vi "For Testing.vi"() -> ()   [LabVIEW 2018]
uses:
  <vilib>/DAQmx/write.llb/DAQmx Write (Analog DBL 1Chan 1Samp).vi
  <vilib>/DAQmx/read.llb/DAQmx Read (Analog DBL 1Chan 1Samp).vi
  <vilib>/addons/control/pid/pid.llb/PID Gain Schedule (DBL).vi
  <vilib>/addons/control/pid/pid.llb/PID Advanced (DBL).vi
  <vilib>/DAQmx/create/channels.llb/DAQmx Create Channel (AI-Voltage-Basic).vi
  <vilib>/DAQmx/miscellaneous.llb/DAQmx Fill In Error Info.vi
  <vilib>/addons/control/pid/NI_PID_pid.lvlib
panel:
  out "Pressure (in torr)":dbl
  out "Scaled MV":dbl(slide) scale=0.0..2000.0
  in  "stop":bool
  out "Preessure Readout":dbl(knob) scale=0.0..1000.0
  in  "Target pressure":dbl
  in  "Sampling Time dt (s)":dbl=0.05 min=0.001 step=0.01 format="%#.3p"
  in  "PID gain schedule":T1(array[cluster])=[{"PID gains"={"proportional gain (Kc)"=1.0, "integral time (Ti, min)"=0.01, "derivative time (Td, min)"=0.0}, "max value"=100.0}] {"max value" format="%.2f"; "PID gains"."derivative time (Td, min)" format="%.6f"; "PID gains"."integral time (Ti, min)" format="%.6f"; "PID gains"."proportional gain (Kc)" format="%.6f"}
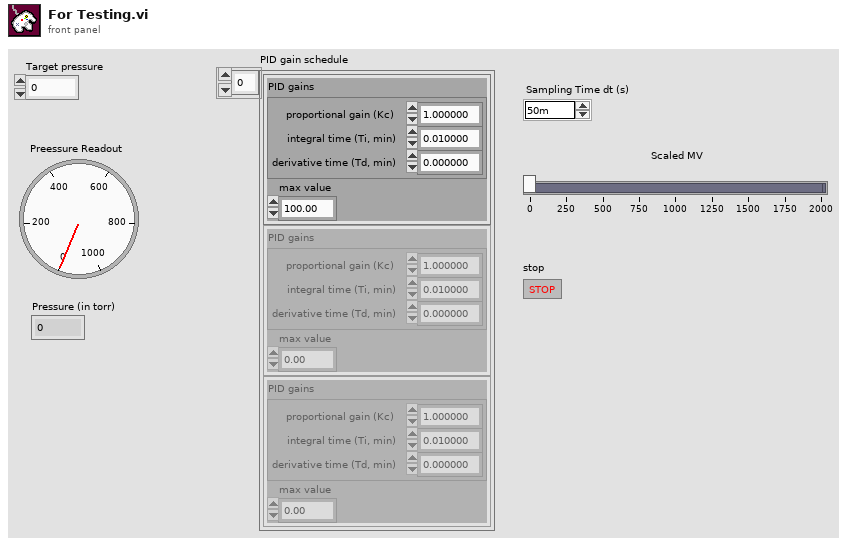
[diagram p1: front panel]
types:
  T1 = cluster{"PID gains":cluster{"proportional gain (Kc)":dbl, "integral time (Ti, min)":dbl, "derivative time (Td, min)":dbl}, "max value":dbl}[]
  T2 = cluster{"proportional gain (Kc)":dbl, "integral time (Ti, min)":dbl, "derivative time (Td, min)":dbl}
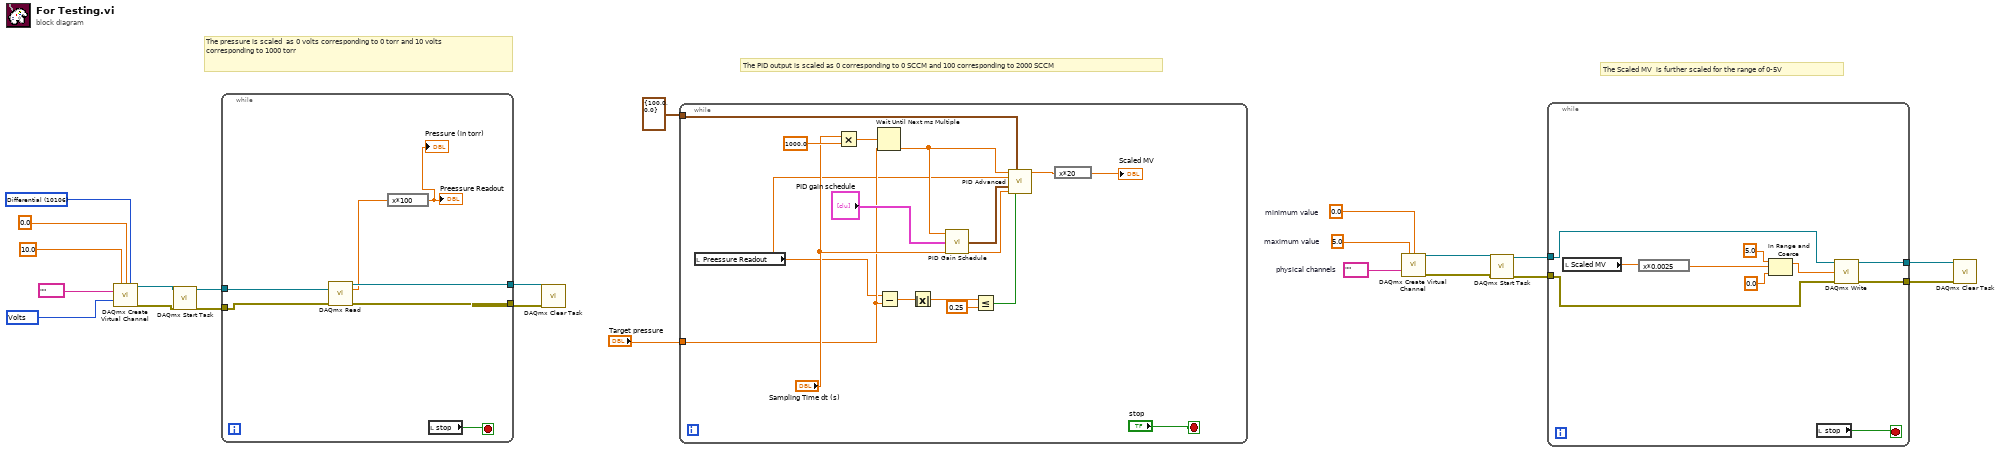
[diagram p0: block diagram]
diagram:
  w3 = tag ""  # physical channels
  w4 = 0.0  # minimum value
  w5 = 5.0  # maximum value
  w10 = 10348 items=["Volts"=10348, "From Custom Scale"=10065] ("units")
  w12 = 10106 items=["Default"=-1, "RSE"=10083, "NRSE"=10078, "Differential"=10106, "Pseudodifferential"=12529] ("input terminal configuration")
  # "The Scaled MV  is further scaled for the range of 0-5V"
  # "The PID output is scaled as 0 corresponding to 0 SCCM and 100 corresponding to 2000 SCCM"
  # "The pressure is scaled  as 0 volts corresponding to 0 torr and 10 volts corresponding to 1000 torr"
  n1 = call-poly <vilib>:"DAQmx Create Virtual Channel.vi"("maximum value"=10.0, "minimum value"=0.0, "input terminal configuration"=w12, "physical channels"=tag "", "units"=w10) -> ("task out"=w20:refnum<k21>, "error out"=w19:errorcluster)  [unwired: 9 in]
  n2 = call <vilib>:"DAQmx Start Task.vi"("task/channels in"=w20, "error in"=w19) -> ("task out"=w18:refnum<k21>, "error out"=w16:errorcluster)  [unwired: 12 in]
  n3 = while {
    tunnel: w18 -> [w29]
    tunnel: [w28] -> w17
    tunnel: w16 -> [w27]
    tunnel: [w26] -> w15
    stop <- w24 stop-if-true
    n4 = call-poly <vilib>:"DAQmx Read.vi"("task/channels in"=w29, "error in"=w27) -> ("task out"=w28:refnum<k21>, "data"=w25:dbl, "error out"=w26:errorcluster)  [unwired: 11 in]
    n5 = expression code="x*100"(w25) -> (→"Preessure Readout" →"Pressure (in torr)":dbl)
    n6 = local read "stop"() -> (w24:bool)
  }
  n7 = call <vilib>:"DAQmx Clear Task.vi"("task in"=w17, "error in"=w15) -> ()  [unwired: 13 in, 1 out]
  n8 = while {
    tunnel: "Target pressure" -> [w35]
    tunnel: cluster{"output high":dbl, "output low":dbl} {"output high"=100.0, "output low"=0.0} ("output range") -> [w34]
    stop <- "stop" stop-if-true
    n9 = local read "Preessure Readout"() -> (w33:dbl)
    n10 = Multiply(x="Sampling Time dt (s)", y=1000.0) -> (x*y=w42:dbl)
    n11 = Wait Until Next ms Multiple(millisecond multiple=w42) -> ()  [unwired: 1 out]
    n12 = Subtract(x=w33, y=w35) -> (x-y=w39:dbl)
    n13 = Absolute Value(x=w39) -> (abs(x)=w38:dbl)
    n14 = call-poly <vilib>:"PID Gain Schedule.vi"("PID gain schedule"="PID gain schedule", "gain scheduling value"=w35) -> ("PID gains out"=w44:T2)  [unwired: 2 in, 1 out]
    n15 = Less Or Equal?(x=w38, y=0.25) -> (x <= y?=w36:bool)
    n16 = call-poly <vilib>:"PID Advanced.vi"("setpoint"=w35, "output range"=w34, "process variable"=w33, "PID gains"=w44, "dt (s)"="Sampling Time dt (s)", "reinitialize? (F)"=w36) -> ("output"=w30:dbl)  [unwired: 8 in, 1 out]
    n17 = expression code="x*20"(w30) -> (→"Scaled MV":dbl)
  }
  n18 = call-poly <vilib>:"DAQmx Create Virtual Channel.vi"("maximum value"=w5, "minimum value"=w4, "physical channels"=w3) -> ("task out"=w7:refnum<k21>, "error out"=w6:errorcluster)  [unwired: 11 in]
  n19 = call <vilib>:"DAQmx Start Task.vi"("task/channels in"=w7, "error in"=w6) -> ("task out"=w2:refnum<k21>, "error out"=w1:errorcluster)  [unwired: 12 in]
  n20 = while {
    tunnel: [w54] -> w9
    tunnel: [w53] -> w8
    tunnel: w2 -> [w48]
    tunnel: w1 -> [w47]
    stop <- w45 stop-if-true
    n21 = local read "Scaled MV"() -> (w46:dbl)
    n22 = expression code="x*0.0025"(w46) -> (w51:dbl)
    n23 = In Range and Coerce(upper limit=5.0, x=w51, lower limit=0.0) -> (coerced(x)=w52:dbl)  [unwired: 1 out]
    n24 = local read "stop"() -> (w45:bool)
    n25 = call-poly <vilib>:"DAQmx Write.vi"("task/channels in"=w48, "data"=w52, "error in"=w47) -> ("task out"=w54:refnum<k21>, "error out"=w53:errorcluster)  [unwired: 10 in, 1 out]
  }
  n26 = call <vilib>:"DAQmx Clear Task.vi"("task in"=w9, "error in"=w8) -> ()  [unwired: 13 in, 1 out]
